vi "RGA queue msg handler (SubVI).vi"(4 "is_running bool":refnum<vi>, 5 "binding key":string, 6 "queue in":refnum<queue>, 8 "error in (no error)":errorcluster, 9 "Exchange.lvclass":refnum<class "Exchange.lvclass">, 10 "log queue in":refnum<queue>, 11 "Queue in":refnum<class "Queue.lvclass">) -> (0 "error out":errorcluster)   [LabVIEW 2016]
uses:
  <vilib>/Distrio/LabbitMQ/Exchange/Exchange.lvclass
  <vilib>/Distrio/LabbitMQ/Queue/Queue.lvclass
  C:/Program Files (x86)/National Instruments/LabVIEW 2016/vi.lib/Distrio/LabbitMQ/RabbitMQ.Client.dll
  Program Files (x86)/National Instruments/LabVIEW 2016/vi.lib/Distrio/LabbitMQ/RabbitMQ.Client.dll
panel:
  out "sent message":string
  in  "stop bool":refnum<vi>
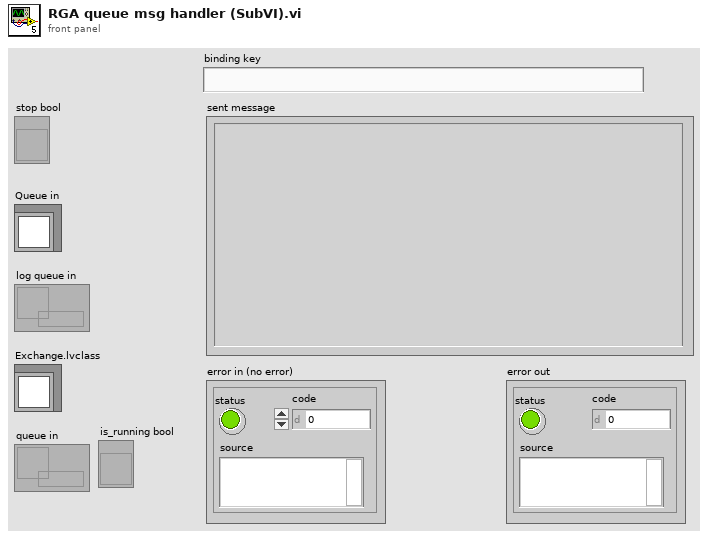
[diagram p1: front panel]
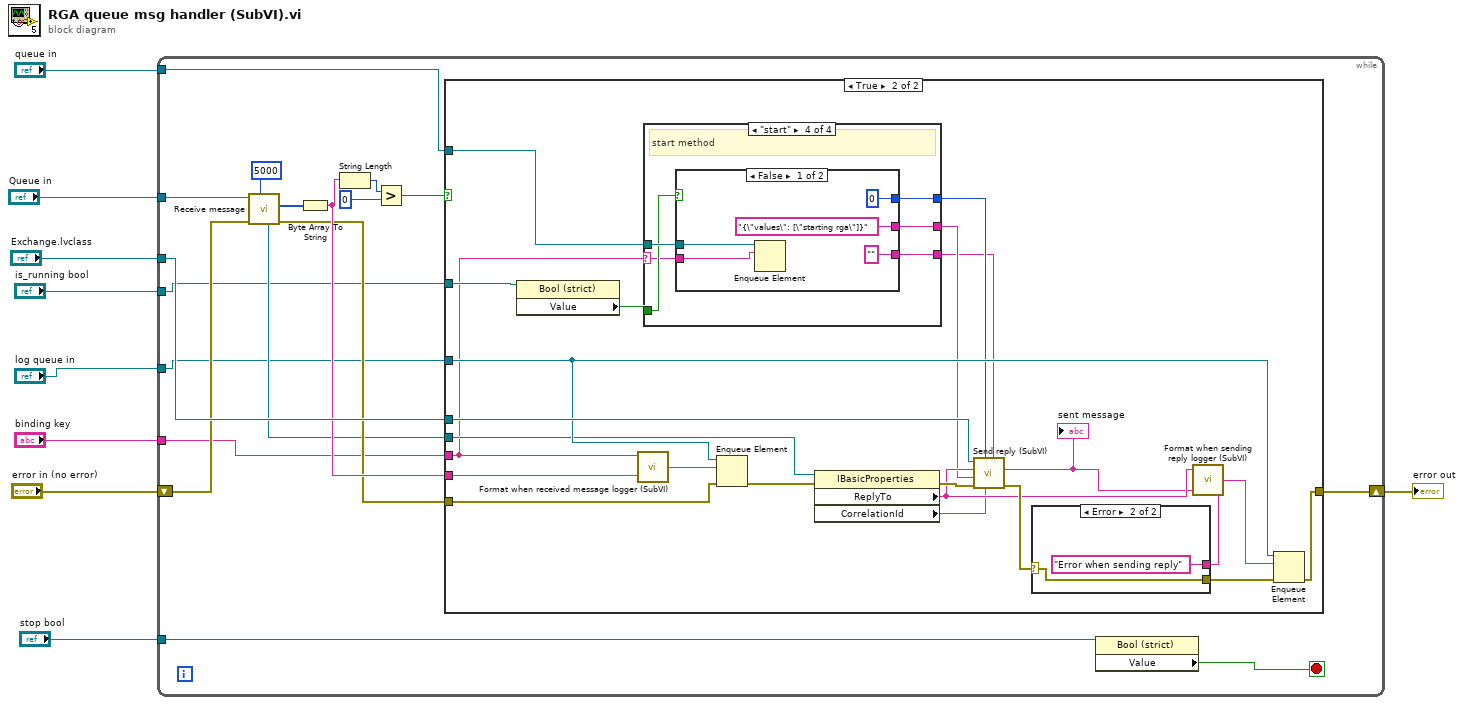
[diagram p0: block diagram]
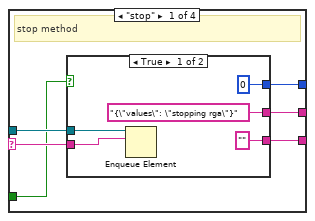
[diagram p3: hidden frame]
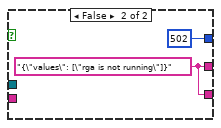
[diagram p4: hidden frame]
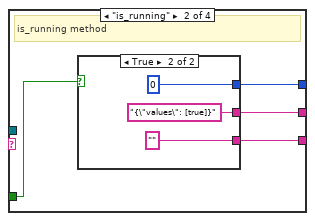
[diagram p5: hidden frame]
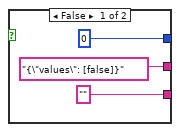
[diagram p6: hidden frame]
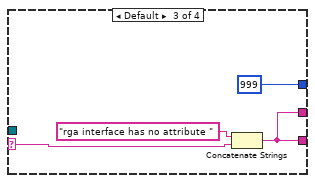
[diagram p7: hidden frame]
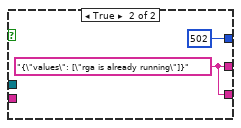
[diagram p8: hidden frame]
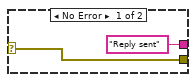
[diagram p9: hidden frame]
diagram:
  n1 = while {
    tunnel: "Exchange.lvclass" -> [w25]
    tunnel: "Queue in" -> [w23]
    tunnel: "is_running bool" -> [w15]
    tunnel: "binding key" -> [w14]
    tunnel: "log queue in" -> [w13]
    tunnel: "queue in" -> [w12]
    shift-right: [w27] -> w9
    shift-left: "error in (no error)" -> [w24]
    tunnel: "stop bool" -> [w11]
    stop <- w10 stop-if-true
    n2 = call <vilib>:"Receive message.vi"("millisecondsTimeout"=5000, "error in (no error)"=w24, "Consumer in"=w23) -> ("error out"=w18:errorcluster, "message body"=w16:u8[], "MessageProperties"=w17:refnum<k24>)  [unwired: 3 in, 3 out]
    n3 = Byte Array To String(unsigned byte array=w16) -> (string=w22:string)
    n4 = String Length(string=w22) -> (length=w19:i32)
    n5 = Greater?(x=w19, y=0) -> (0:w21:bool)
    n6 = case shown="True" w21 {
      tunnel: w17 -> [_ w42]
      tunnel: w22 -> [_ w51]
      tunnel: w18 -> [w28 w40]
      tunnel: [w28 w44] -> w27
      tunnel: w25 -> [_ w50]
      tunnel: w12 -> [_ w49]
      tunnel: w13 -> [_ w46]
      tunnel: w14 -> [_ w30]
      tunnel: w15 -> [_ w32]
      frame False {
      }
      frame True {
        n7 = property class="Bool (strict)"(reference=w32) -> ("Value"=w31:bool)  [unwired: 1 in, 2 out]
        n8 = call "Format when received message logger (SubVI).vi"("received message"=w51, "queue name"=w30) -> ("info to log"=w48:string)
        n9 = case shown="\"start\"" w30 {
          selector: w30 -> [w57 _ w76 w81]
          tunnel: w49 -> [w56 _ _ w84]
          tunnel: [w54 w67 w75 w83] -> w35
          tunnel: w31 -> [w55 w68 _ w82]
          tunnel: [w53 w66 999 w80] -> w34
          tunnel: [w52 w65 w75 w79] -> w33
          frame "stop" {
            # "stop method"
            n10 = case shown="True" w55 {
              tunnel: w56 -> [w62 _]
              tunnel: ["{\"values\": \"stopping rga\"}" ("reply content if running") w64] -> w54
              tunnel: w57 -> [w60 _]
              tunnel: [0 502] -> w53
              tunnel: ["" ("reply content if running") w64] -> w52
              frame True {
                n11 = Enqueue Element(queue=w62, element=w60) -> ()  [unwired: 2 in, 3 out]
              }
              frame False {
                w64 = "{\"values\": [\"rga is not running\"]}" ("reply content if running")
              }
            }
          }
          frame "is_running" {
            # "is_running method"
            n12 = case shown="True" w68 {
              tunnel: ["{\"values\": [false]}" "{\"values\": [true]}"] -> w67
              tunnel: [0 0] -> w66
              tunnel: ["" ""] -> w65
              frame False {
              }
              frame True {
              }
            }
          }
          frame Default {
            n13 = Concatenate Strings("rga interface has no attribute " ("reply content if running"), w76) -> (w75:string)
          }
          frame "start" {
            # "start method"
            n14 = case shown="False" w82 {
              tunnel: w84 -> [w89 _]
              tunnel: ["{\"values\": [\"starting rga\"]}" ("reply content if running") w91] -> w83
              tunnel: w81 -> [w87 _]
              tunnel: [0 502] -> w80
              tunnel: ["" ("reply content if running") w91] -> w79
              frame False {
                n15 = Enqueue Element(queue=w89, element=w87) -> ()  [unwired: 2 in, 3 out]
              }
              frame True {
                w91 = "{\"values\": [\"rga is already running\"]}" ("reply content if running")
              }
            }
          }
        }
        n16 = Enqueue Element(queue=w46, element=w48, error in (no error)=w40) -> (error out=w39:errorcluster)  [unwired: 1 in, 2 out]
        n17 = property class="IBasicProperties"(reference=w42, error in=w39) -> (error out=w41:errorcluster, "ReplyTo"=w38:string, "CorrelationId"=w37:string)  [unwired: 1 out]
        n18 = call "Send reply (SubVI).vi"("return_msg"=w33, "Correlation ID"=w37, "retcode"=w34, "error in (no error)"=w41, "reply content"=w35, "target"=w38, "Exchange.lvclass"=w50) -> ("error out"=w45:errorcluster, "sent message"=w36:string)  [unwired: 3 in]
        "sent message" <- w36
        n19 = case shown="Error" w45 {
          selector: w45 -> [w92 w94]
          tunnel: ["Reply sent" ("string") "Error when sending reply" ("string")] -> w47
          tunnel: [w92 w94] -> w29
          frame No Error {
          }
          frame Error {
          }
        }
        n20 = call "Format when sending reply logger (SubVI).vi"("sent message"=w36, "status"=w47, "queue name"=w38) -> ("info to log"=w43:string)
        n21 = Enqueue Element(queue=w46, element=w43, error in (no error)=w29) -> (error out=w44:errorcluster)  [unwired: 1 in, 2 out]
      }
    }
    n22 = property class="Bool (strict)"(reference=w11) -> ("Value"=w10:bool)  [unwired: 1 in, 2 out]
  }
  "error out" <- w9
